vi "Splash.vi"() -> ()   [LabVIEW 2020]
panel:
  out "Imaging  VI Path":path=path "E:/Norway Project/All Hardware/New Microscope/LabVIEW/H5ViewerSAM/DataView.vi"
  out "Analysis  VI Path":path=path "E:/Norway Project/All Hardware/New Microscope/LabVIEW/H5ViewerSAM/DataView.vi"
  in  "Quit Button":bool
  in  "Imaging Button":bool
  in  "Analysis Button":bool
  # "Developed By Prakhar Kumar (pka.alld.97@gmail.com)"
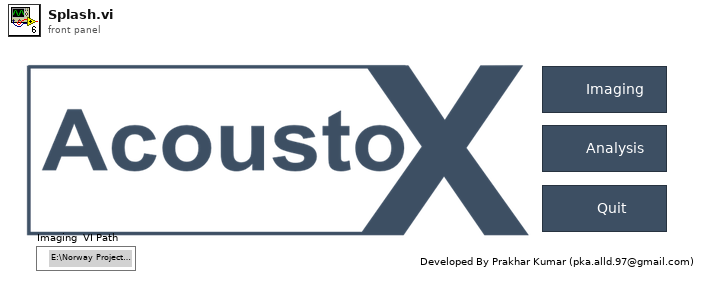
[diagram p1: front panel]
types:
  T1 = enum32{"Invalid", "Standard", "Closed", "Hidden", "Minimized", "Maximized"}
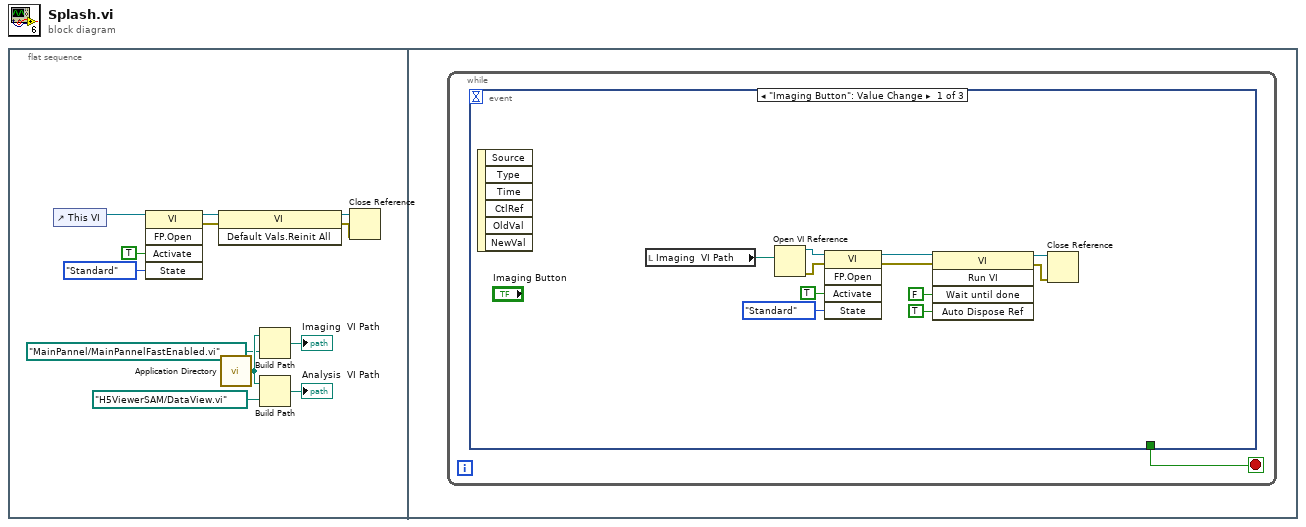
[diagram p0: block diagram]
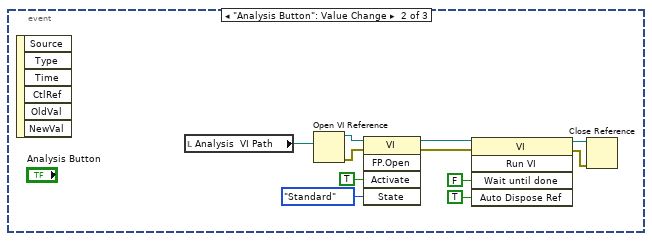
[diagram p2: hidden frame]
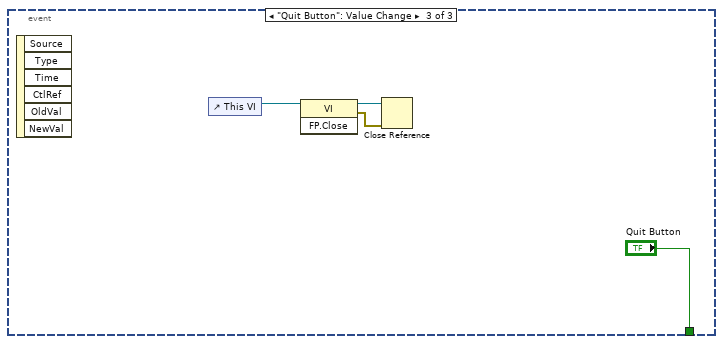
[diagram p3: hidden frame]
diagram:
  n1 = flat-sequence {
    frame #0 {
      n2 = control-ref of="This VI"() -> (w12:refnum<vi>)
      n3 = invoke class="VI" method="FP.Open"(reference=w12, "Activate"=TRUE ("Activate?"), "State"=T1."Standard") -> (reference out=w9:refnum<vi>, error out=w8:errorcluster)  [unwired: 2 in, 3 out]
      n4 = invoke class="VI" method="Default Vals.Reinit All"(reference=w9, error in=w8) -> (reference out=w6:refnum<vi>, error out=w7:errorcluster)  [unwired: 1 in, 1 out]
      n5 = call <vilib>:"Application Directory.vi"() -> ("Application Directory"=w4:path)
      n6 = Build Path(base path=w4, name or relative path=path "MainPannel/MainPannelFastEnabled.vi" ("vi path")) -> (appended path=→"Imaging  VI Path":path)
      n7 = Build Path(base path=w4, name or relative path=path "H5ViewerSAM/DataView.vi" ("vi path")) -> (appended path=→"Analysis  VI Path":path)
      n8 = Close Reference(reference=w6, error in (no error)=w7) -> ()  [unwired: 1 out]
    }
    frame #1 {
      n9 = while {
        stop <- w13 stop-if-true
        n10 = event shown="[0] \"Imaging Button\": Value Change" {
          selector: _ -> [_ _ _]
          dyn-events: _ -> [_ _ _]
          timeout: _ -> [_ _ _]
          tunnel: [_ _ "Quit Button"] -> w13
          event "Imaging Button": Value Change {
            n11 = event-data() -> ()  [unwired: 1 in, 6 out]
            n12 = local read "Imaging  VI Path"() -> (w24:path)
            n13 = Open VI Reference(vi path=w24) -> (vi reference=w23:refnum<vi>, error out=w22:errorcluster)  [unwired: 5 in]
            n14 = invoke class="VI" method="FP.Open"(reference=w23, error in=w22, "Activate"=TRUE ("Activate?"), "State"=T1."Standard") -> (reference out=w19:refnum<vi>, error out=w18:errorcluster)  [unwired: 1 in, 3 out]
            n15 = invoke class="VI" method="Run VI"(reference=w19, error in=w18, "Wait until done"=FALSE ("Wait Until Done"), "Auto Dispose Ref"=TRUE ("Auto Dispose Reference")) -> (reference out=w15:refnum<vi>, error out=w14:errorcluster)  [unwired: 1 in, 3 out]
            n16 = Close Reference(reference=w15, error in (no error)=w14) -> ()  [unwired: 1 out]
          }
          event "Analysis Button": Value Change {
            n17 = event-data() -> ()  [unwired: 1 in, 6 out]
            n18 = local read "Analysis  VI Path"() -> (w35:path)
            n19 = Open VI Reference(vi path=w35) -> (vi reference=w34:refnum<vi>, error out=w33:errorcluster)  [unwired: 5 in]
            n20 = invoke class="VI" method="FP.Open"(reference=w34, error in=w33, "Activate"=TRUE ("Activate?"), "State"=T1."Standard") -> (reference out=w30:refnum<vi>, error out=w29:errorcluster)  [unwired: 1 in, 3 out]
            n21 = invoke class="VI" method="Run VI"(reference=w30, error in=w29, "Wait until done"=FALSE ("Wait Until Done"), "Auto Dispose Ref"=TRUE ("Auto Dispose Reference")) -> (reference out=w26:refnum<vi>, error out=w25:errorcluster)  [unwired: 1 in, 3 out]
            n22 = Close Reference(reference=w26, error in (no error)=w25) -> ()  [unwired: 1 out]
          }
          event "Quit Button": Value Change {
            n23 = event-data() -> ()  [unwired: 1 in, 6 out]
            n24 = control-ref of="This VI"() -> (w38:refnum<vi>)
            n25 = invoke class="VI" method="FP.Close"(reference=w38) -> (reference out=w37:refnum<vi>, error out=w36:errorcluster)  [unwired: 2 in, 1 out]
            n26 = Close Reference(reference=w37, error in (no error)=w36) -> ()  [unwired: 1 out]
          }
        }
      }
    }
  }
